vi "Lin_Rohner_force_sensor_tachometer.vi"() -> ()   [LabVIEW 2019]
uses:
  <vilib>/Platform/TimedLoop/XDataNode/timing_clust.ctl
  <vilib>/Platform/TimedLoop/XDataNode/nitl_modes.ctl
  <vilib>/Platform/TimedLoop/XDataNode/wakeup.ctl
  <vilib>/Analysis/3filter.llb/Filter Passband Type.ctl
  <vilib>/DAQmx/write.llb/DAQmx Write (Analog DBL 1Chan 1Samp).vi
  <vilib>/DAQmx/read.llb/DAQmx Read (Analog 1D DBL NChan 1Samp).vi
  <vilib>/DAQmx/create/channels.llb/DAQmx Create Channel (AI-Voltage-Basic).vi
  <vilib>/DAQmx/create/channels.llb/DAQmx Create Channel (AO-Voltage-Basic).vi
  <vilib>/DAQmx/miscellaneous.llb/DAQmx Fill In Error Info.vi
  <vilib>/platform/TimedLoop/XDataNode/XDataNode.xnode
  <vilib>/Platform/TimedLoop/XDataNode/XDNodeRunTimeDep.lvlib
  <vilib>/ptbypt/NI_PtbyPt.lvlib
  <vilib>/Analysis/NI_AALBase.lvlib
panel:
  in  "low cutoff freq: paddle angular velocity(tachometer) 2":dbl=0.125 format="%0.3f"
  out "Raw Paddle Angular Acce(tachometer) [rad/s^2]":dbl(graph)
  out "Raw Paddle Angular Acce(tachometer) [rad/s^2]":dbl
  out "Filtered Paddle Angular Velocity(tachometer) [rad/s]":dbl
  out "Filtered Paddle Angular Velocity(tachometer) [rad/s]":dbl(graph)
  in  "low cutoff freq: paddle angular velocity(tachometer)":dbl=0.125 format="%0.3f"
  out "Raw Force [N]":dbl
  out "Raw Force [N]":dbl(graph)
  out "Filtered Paddle Angular Velocity(derivative) [rad/s]":dbl
  out "Filtered Paddle Angular Velocity(derivative) [rad/s]":dbl(graph)
  in  "low cutoff freq: angular velocity(derivative)":dbl=0.125 format="%0.3f"
  out "Raw Paddle Angular Velocity(tachometer) [rad/s]":dbl
  out "Raw Paddle Angular Velocity(tachometer) [rad/s]":dbl(graph)
  out "Raw Tachometer[V]":dbl
  out "Raw Tachometer[V]":dbl(graph)
  out "Filtered Force Sensor [V]":dbl
  out "Filtered Force Sensor [V]":dbl(graph)
  in  "low cutoff freq: force sensor)":dbl=0.125 format="%0.3f"
  out "Raw Force sensor [V]":dbl
  out "Raw Force sensor [V]":dbl(graph)
  out "Position [deg]":dbl(knob) scale=-32.5..32.5
  out "Filtered Position [deg]":dbl
  out "Filtered Postion Graph [deg]":dbl(graph)
  in  "stop":bool
  in  "low cutoff freq: position":dbl=0.125 format="%0.3f"
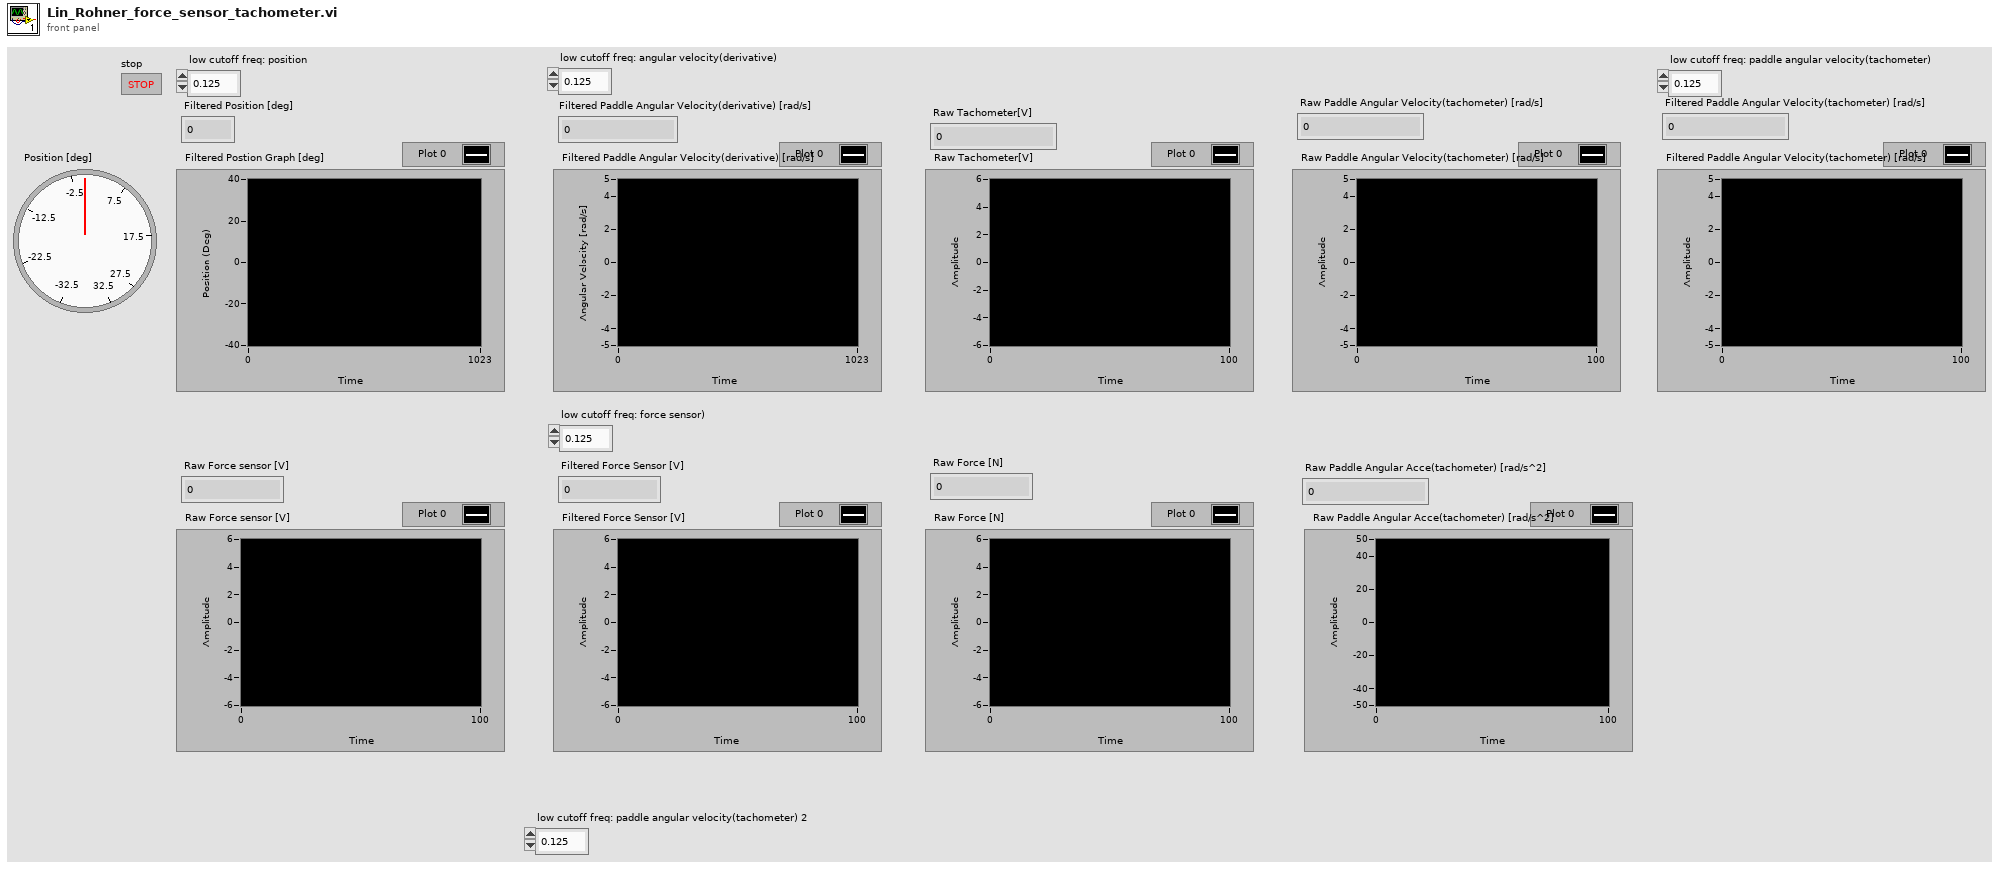
[diagram p1: front panel]
types:
  T1 = typedef "NI_AALBase.lvlib/Filter Passband Type.ctl" = enum32{"Lowpass", "Highpass", "Bandpass", "Bandstop"}
  T2 = typedef "XDNodeRunTimeDep.lvlib/timing_clust.ctl" = cluster{"Expected End [f-1]":u64, "Actual End [f-1]":u64, "Finished Late? [f-1]":bool, "Expected End [i-1]":u64, "Actual End [i-1]":u64, "Finished Late? [i-1]":bool, "Expected Start [i]":u64, "Actual Start [i]":u64, "Expected Start [f]":u64, "Actual Start [f]":u64, "Source Name":string, "Structure Name":string, "Period":i64, "Deadline":i64, "Offset":i64, "Start":i64, "Priority":i32, "Timeout":i32, "Mode":T3, "Wakeup Reason":T4, "Error":errorcluster, "Source Type":string, "Secondary Source Type":string, "Global End Time":u64, "Global Start Time":u64, "Frame Duration":u64, "Iteration Duration":u64, "Assigned CPU":i32, "I/O Scan Engine Mode":u32}
  T3 = typedef "XDNodeRunTimeDep.lvlib/nitl_modes.ctl" = enum32{"No Change", "Process missed periods, maintain original phase", "Discard missed periods, maintain original phase", "Process missed periods, ignore original phase", "Discard missed periods, ignore original phase"}
  T4 = typedef "XDNodeRunTimeDep.lvlib/wakeup.ctl" = enum32{"Normal", "Aborted", "Asynchronous wakeup", "Timing source error", "Timed loop error", "Timeout"}
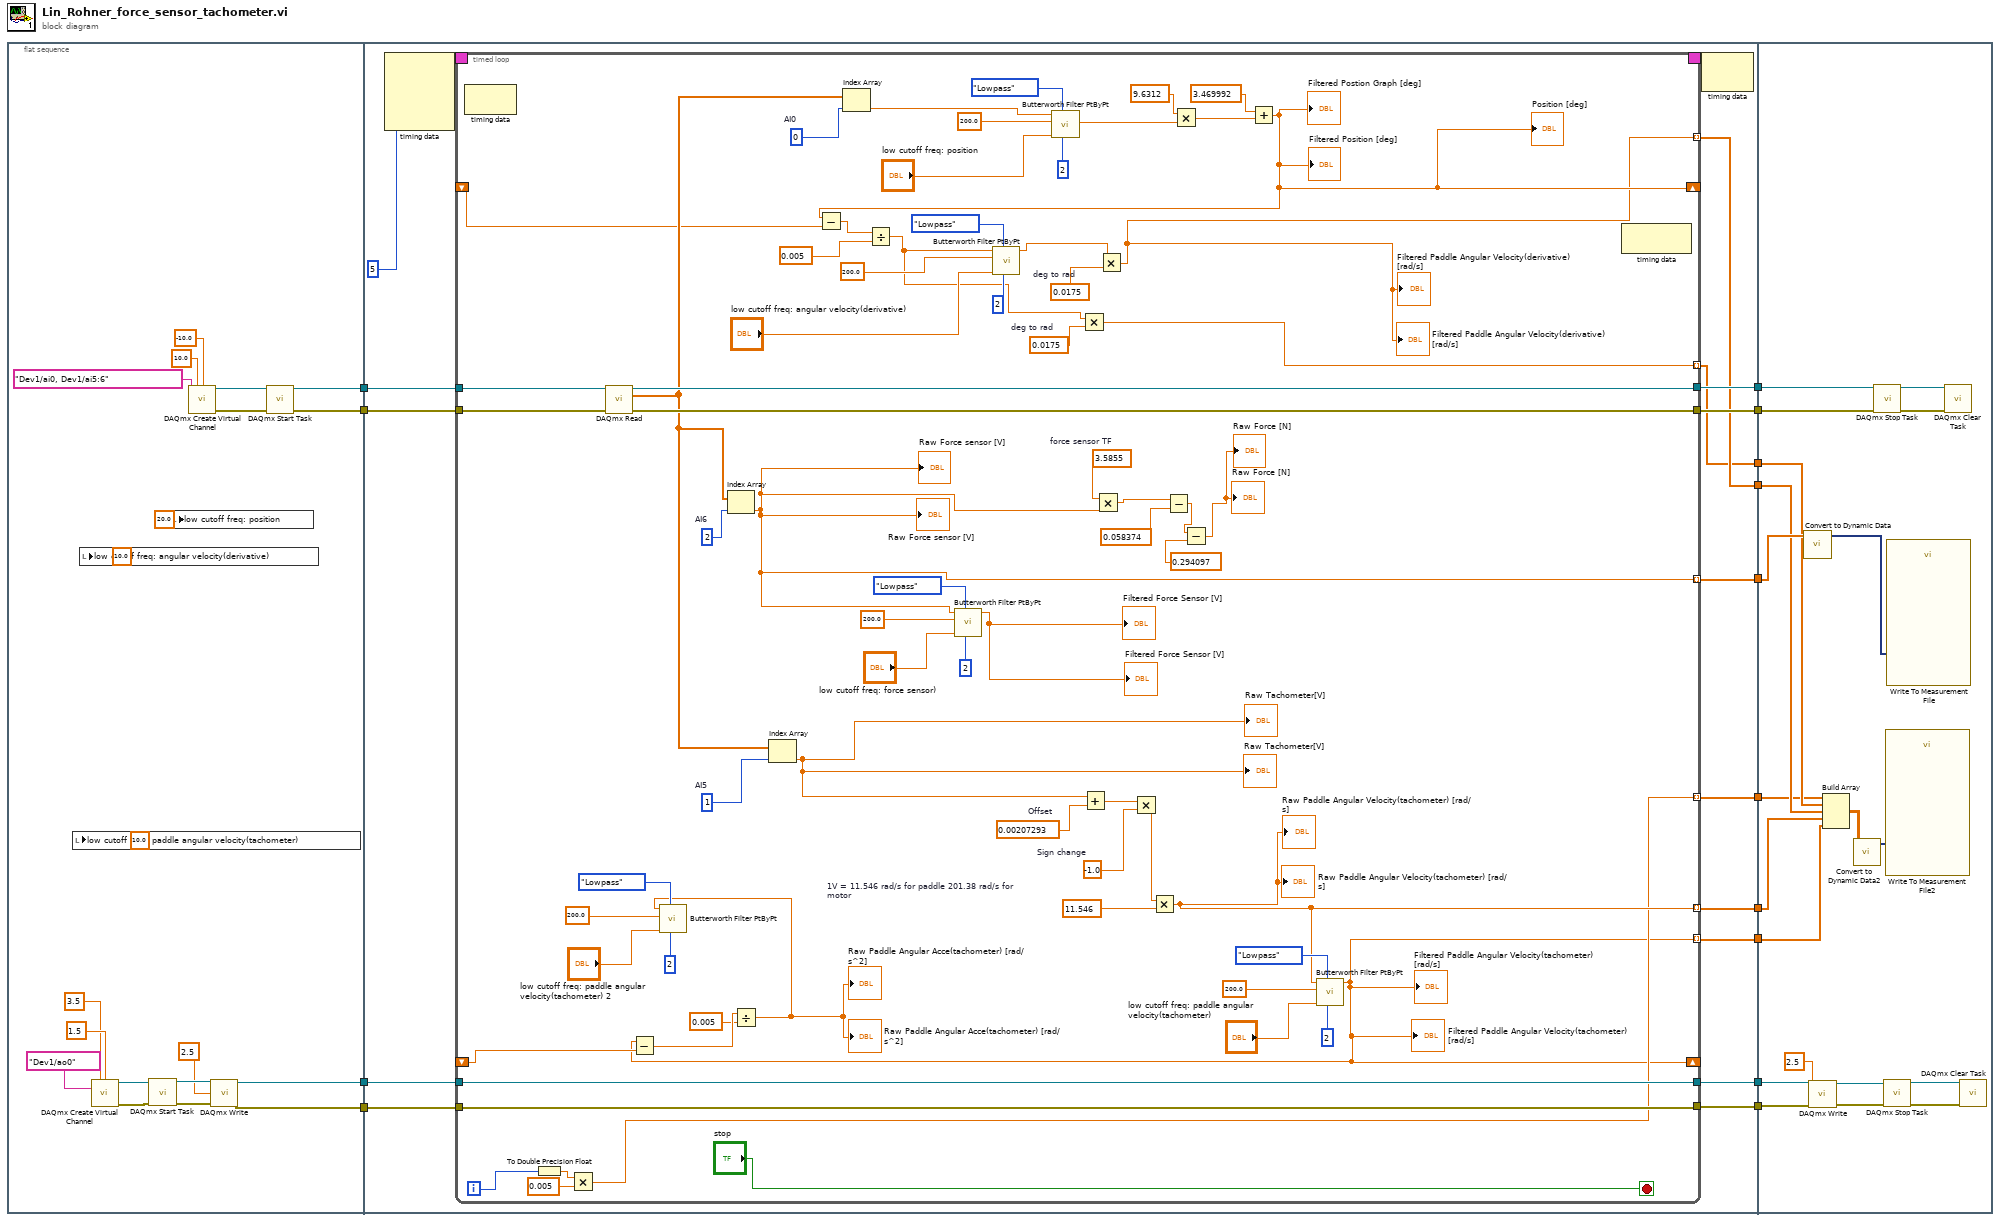
[diagram p0: block diagram]
diagram:
  n1 = flat-sequence {
    tunnel: [w31] -> w14
    tunnel: [w29] -> w12
    tunnel: [w19] -> w9
    tunnel: [w18] -> w8
    tunnel: w14 -> [w49]
    tunnel: [w48] -> w13
    tunnel: w12 -> [w47]
    tunnel: [w46] -> w11
    tunnel: [w44] -> w10
    tunnel: w9 -> [w43]
    tunnel: w8 -> [w42]
    tunnel: [w41] -> w7
    tunnel: [w40] -> w6
    tunnel: [w39] -> w5
    tunnel: [w38] -> w4
    tunnel: [w37] -> w3
    tunnel: [w36] -> w2
    tunnel: [w35] -> w1
    tunnel: w13 -> [w147]
    tunnel: w11 -> [w145]
    tunnel: w10 -> [w143]
    tunnel: w7 -> [w136]
    tunnel: w6 -> [w135]
    tunnel: w5 -> [w134]
    tunnel: w4 -> [w133]
    tunnel: w3 -> [w130]
    tunnel: w2 -> [w129]
    tunnel: w1 -> [w128]
    frame #0 {
      n2 = local write "low cutoff freq: paddle angular velocity(tachometer)"(10.0 ("filter Techometer 2")) -> ()
      n3 = local write "low cutoff freq: angular velocity(derivative)"(10.0 ("low cutoff freq: fl 3")) -> ()
      n4 = call-poly <vilib>:"DAQmx Create Virtual Channel.vi"("maximum value"=3.5, "minimum value"=1.5, "physical channels"=tag "Dev1/ao0") -> ("task out"=w27:refnum<k21>, "error out"=w25:errorcluster)  [unwired: 11 in]
      n5 = call <vilib>:"DAQmx Start Task.vi"("task/channels in"=w27, "error in"=w25) -> ("task out"=w26:refnum<k21>, "error out"=w24:errorcluster)  [unwired: 12 in]
      n6 = local write "low cutoff freq: position"(20.0 ("low cutoff freq: fl 2")) -> ()
      n7 = call-poly <vilib>:"DAQmx Create Virtual Channel.vi"("maximum value"=10.0, "minimum value"=-10.0, "physical channels"=tag "Dev1/ai0, Dev1/ai5:6") -> ("task out"=w30:refnum<k21>, "error out"=w32:errorcluster)  [unwired: 11 in]
      n8 = call-poly <vilib>:"DAQmx Write.vi"("task/channels in"=w26, "data"=2.5, "error in"=w24) -> ("task out"=w19:refnum<k21>, "error out"=w18:errorcluster)  [unwired: 10 in, 1 out]
      n9 = call <vilib>:"DAQmx Start Task.vi"("task/channels in"=w30, "error in"=w32) -> ("task out"=w29:refnum<k21>, "error out"=w31:errorcluster)  [unwired: 12 in]
    }
    frame #1 {
      n10 = node-c288(i64 5 ("Period")) -> (w51:T2)  [unwired: 3 in]
      n11 = timed-loop {
        timing: w51 -> [_]
        timing-out: [_] -> w50
        tunnel: w49 -> [w121]
        tunnel: [w120] -> w48
        tunnel: w47 -> [w116]
        tunnel: [w115] -> w46
        tunnel: [w80] -> w44 mode=indexing
        tunnel: w43 -> [w98]
        tunnel: w42 -> [w97]
        tunnel: [w98] -> w41
        tunnel: [w97] -> w40
        shift-right: [w90] -> _
        shift-left: _ -> [w89]
        tunnel: [w72] -> w39 mode=indexing
        tunnel: [w59] -> w38 mode=indexing
        tunnel: [w71] -> w37 mode=indexing
        tunnel: [w64] -> w36 mode=indexing
        tunnel: [w67] -> w35 mode=indexing
        shift-right: [w59] -> _
        shift-left: _ -> [w60]
        i -> [w70]
        stop <- "stop" stop-if-true
        w65 = 0.0175  # deg to rad
        w79 = 3.5855  # force sensor TF
        w81 = 0.0175  # deg to rad
        w91 = 11.546  # 1V = 11.546 rad/s for paddle 201.38 rad/s for motor
        w93 = -1.0  # Sign change
        w95 = 0.00207293  # Offset
        w99 = 1  # AI5
        w106 = 2  # AI6
        w108 = 0  # AI0
        n12 = node-c288() -> ()  [unwired: 1 in, 1 out]
        n13 = To Double Precision Float(number=w70) -> (double precision float=w69:dbl)
        n14 = Multiply(x=w69, y=0.005) -> (x*y=w67:dbl)
        n15 = call-poly <vilib>:"DAQmx Read.vi"("task/channels in"=w116, "error in"=w121) -> ("task out"=w115:refnum<k21>, "data"=w100:dbl[], "error out"=w120:errorcluster)  [unwired: 11 in]
        n16 = Index Array(array=w100, index=w106) -> (element=w80:dbl)
        "Raw Force sensor [V]" <- w80
        "Raw Force sensor [V]" <- w80
        n17 = Index Array(array=w100, index=w99) -> (element=w96:dbl)
        "Raw Tachometer[V]" <- w96
        "Raw Tachometer[V]" <- w96
        n18 = Index Array(array=w100, index=w108) -> (element=w107:dbl)
        n19 = call <vilib>:"Butterworth Filter PtByPt.vi"("order"=2, "filter type"=Filter_Passband_Type."Lowpass", "low cutoff freq: fl"="low cutoff freq: force sensor)", "sampling freq: fs"=200.0, "x"=w80) -> ("Filtered x"=→"Filtered Force Sensor [V]" →"Filtered Force Sensor [V]":dbl)  [unwired: 4 in, 1 out]
        n20 = call <vilib>:"Butterworth Filter PtByPt.vi"("order"=2, "filter type"=Filter_Passband_Type."Lowpass", "low cutoff freq: fl"="low cutoff freq: position", "sampling freq: fs"=200.0, "x"=w107) -> ("Filtered x"=w109:dbl)  [unwired: 4 in, 1 out]
        n21 = Add(x=w96, y=w95) -> (x+y=w94:dbl)
        n22 = Multiply(x=w79, y=w80) -> (x*y=w78:dbl)
        n23 = Multiply(x=w94, y=w93) -> (x*y=w92:dbl)
        n24 = Multiply(x=w92, y=w91) -> (x*y=w72:dbl)
        "Raw Paddle Angular Velocity(tachometer) [rad/s]" <- w72
        "Raw Paddle Angular Velocity(tachometer) [rad/s]" <- w72
        n25 = Subtract(x=w78, y=0.058374) -> (x-y=w62:dbl)
        n26 = Multiply(x=9.6312, y=w109) -> (x*y=w111:dbl)
        n27 = Subtract(x=w62, y=0.294097) -> (x-y=→"Raw Force [N]" →"Raw Force [N]":dbl)
        n28 = Add(x=3.469992, y=w111) -> (x+y=w90:dbl)
        "Filtered Postion Graph [deg]" <- w90
        "Filtered Position [deg]" <- w90
        "Position [deg]" <- w90
        n29 = Subtract(x=w90, y=w89) -> (x-y=w88:dbl)
        n30 = Divide(x=w88, y=0.005) -> (x/y=w66:dbl)
        n31 = call <vilib>:"Butterworth Filter PtByPt.vi"("order"=2, "filter type"=Filter_Passband_Type."Lowpass", "low cutoff freq: fl"="low cutoff freq: angular velocity(derivative)", "sampling freq: fs"=200.0, "x"=w66) -> ("Filtered x"=w82:dbl)  [unwired: 4 in, 1 out]
        n32 = Multiply(x=w66, y=w65) -> (x*y=w64:dbl)
        n33 = Multiply(x=w82, y=w81) -> (x*y=w71:dbl)
        "Filtered Paddle Angular Velocity(derivative) [rad/s]" <- w71
        "Filtered Paddle Angular Velocity(derivative) [rad/s]" <- w71
        n34 = call <vilib>:"Butterworth Filter PtByPt.vi"("order"=2, "filter type"=Filter_Passband_Type."Lowpass", "low cutoff freq: fl"="low cutoff freq: paddle angular velocity(tachometer)", "sampling freq: fs"=200.0, "x"=w72) -> ("Filtered x"=w59:dbl)  [unwired: 4 in, 1 out]
        "Filtered Paddle Angular Velocity(tachometer) [rad/s]" <- w59
        "Filtered Paddle Angular Velocity(tachometer) [rad/s]" <- w59
        n35 = Subtract(x=w59, y=w60) -> (x-y=w58:dbl)
        n36 = Divide(x=w58, y=0.005) -> (x/y=w52:dbl)
        "Raw Paddle Angular Acce(tachometer) [rad/s^2]" <- w52
        "Raw Paddle Angular Acce(tachometer) [rad/s^2]" <- w52
        n37 = call <vilib>:"Butterworth Filter PtByPt.vi"("order"=2, "filter type"=Filter_Passband_Type."Lowpass", "low cutoff freq: fl"="low cutoff freq: paddle angular velocity(tachometer) 2", "sampling freq: fs"=200.0, "x"=w52) -> ()  [unwired: 4 in, 2 out]
        n38 = node-c288() -> ()  [unwired: 1 in, 1 out]
      }
      n39 = node-c288(w50) -> ()  [unwired: 1 out]
    }
    frame #2 {
      n40 = call "Convert to Dynamic Data"("Array"=w143) -> ("Dynamic Data Type"=w142:dynamicdata)  [unwired: 3 in]
      n41 = call-poly <vilib>:"DAQmx Write.vi"("task/channels in"=w136, "data"=2.5, "error in"=w135) -> ("task out"=w141:refnum<k21>, "error out"=w138:errorcluster)  [unwired: 10 in, 1 out]
      n42 = Build Array(w128, w129, w130, w134, w133) -> (w132:dbl[][])
      n43 = call "Convert to Dynamic Data2"("2D Array"=w132) -> ("Dynamic Data Type"=w131:dynamicdata)  [unwired: 3 in]
      n44 = call <vilib>:"DAQmx Stop Task.vi"("task/channels in"=w145, "error in"=w147) -> ("task out"=w144:refnum<k21>, "error out"=w146:errorcluster)  [unwired: 12 in]
      n45 = call <vilib>:"DAQmx Stop Task.vi"("task/channels in"=w141, "error in"=w138) -> ("task out"=w140:refnum<k21>, "error out"=w139:errorcluster)  [unwired: 12 in]
      n46 = call "Write To Measurement File2"("Signals"=w131) -> ()  [unwired: 16 in, 3 out]
      n47 = call "Write To Measurement File"("Signals"=w142) -> ()  [unwired: 16 in, 3 out]
      n48 = call <vilib>:"DAQmx Clear Task.vi"("task in"=w144, "error in"=w146) -> ()  [unwired: 13 in, 1 out]
      n49 = call <vilib>:"DAQmx Clear Task.vi"("task in"=w140, "error in"=w139) -> ()  [unwired: 13 in, 1 out]
    }
  }
